vi "DAQ_System.vi"() -> ()   [LabVIEW 2023]
doc: "This is the Main VI that performs DAQ system and simulate the Same."
uses:
  Controls/DAQ Inputs.ctl
  Controls/DAQ_Output.ctl
  Controls/Queue_Operation_Select.ctl
  Controls/DAQ_Data.ctl
  Controls/Acquired_Data.ctl
  Controls/State_and_Data.ctl
  Controls/Notifier_Operation_Select.ctl
  Controls/Timer_Select.ctl
  Controls/Error_Data.ctl
panel:
  out "Error_Out":errorcluster
  in  "Error_In":errorcluster
  in  "Stop":bool
  out "DAQ_Output":T1
  in  "DAQ_Inputs":T2={"Digial_In"={"AC_Power_Supply"=FALSE}, "Analog_In"={"Power_Consumption"=0.0, "Battery_Power"=100.0}} caption="DAQ Inputs" {"Analog_In"."Battery_Power" scale=0.0..100.0; "Analog_In"."Power_Consumption" scale=0.0..10.0}
  # "DAQ Simulator"
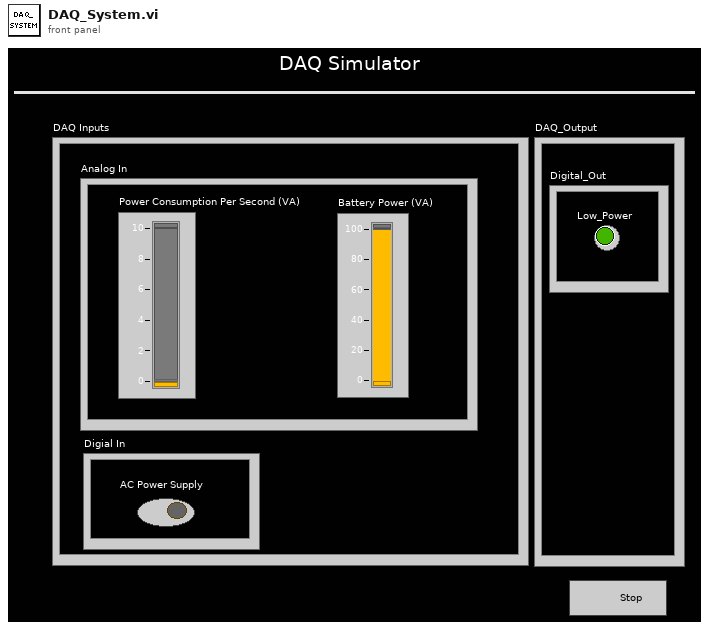
[diagram p1: front panel]
types:
  T1 = typedef "DAQ_Output.ctl" = cluster{"Digital_Out":cluster{"Low_Power":bool}}
  T2 = typedef "DAQ Inputs.ctl" = cluster{"Digial_In":cluster{"AC_Power_Supply":bool}, "Analog_In":cluster{"Power_Consumption":dbl, "Battery_Power":dbl}}
  T3 = typedef "State_and_Data.ctl" = cluster{"State":string, "Data":variant}
  T4 = typedef "Timer_Select.ctl" = enum16{"Start_Timer", "Time_Out?", "Stop_Timer"}
  T5 = typedef "Notifier_Operation_Select.ctl" = enum16{"Obtain_Notifier", "Send_Notification", "Get_Notifier_Status", "Release_Notifier"}
  T6 = typedef "Queue_Operation_Select.ctl" = enum16{"Obtain_Queue", "Enqueue", "Enqueue_First", "Enqueue_N", "Lossy_Enqueue", "Preview", "Queue_Status", "Dequeue", "Flush", "Release_Queue"}
  T7 = typedef "DAQ_Data.ctl" = cluster{"Acquired_Data":T8, "DAQ_Output":T1, "DAQ_Inputs":T2, "Data_In":T3, "Start":bool}
  T8 = typedef "Acquired_Data.ctl" = cluster{"Battery_Power":dbl, "Power_Consumption":dbl, "Inverter_Mode":bool}
  T9 = enum32{"Invalid", "Standard", "Closed", "Hidden", "Minimized", "Maximized"}
  T10 = typedef "Error_Data.ctl" = cluster{"Module_Name":string, "Error":errorcluster}
  T11 = cluster{"Power_Consumption":dbl, "Battery_Power":dbl}
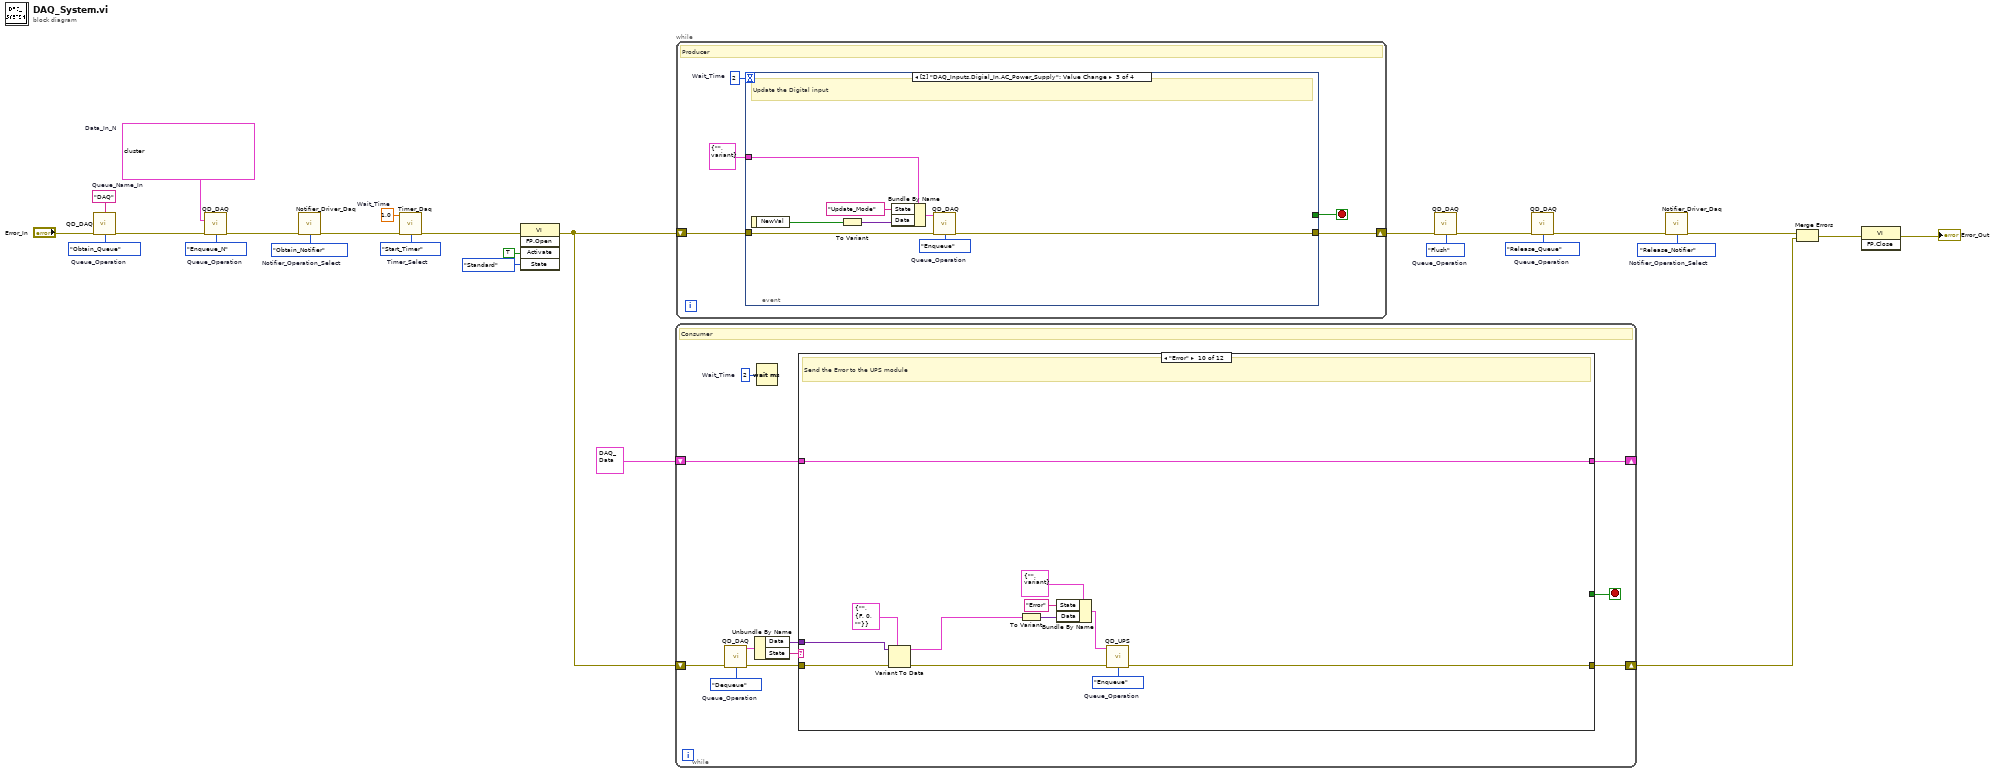
[diagram p0: block diagram]
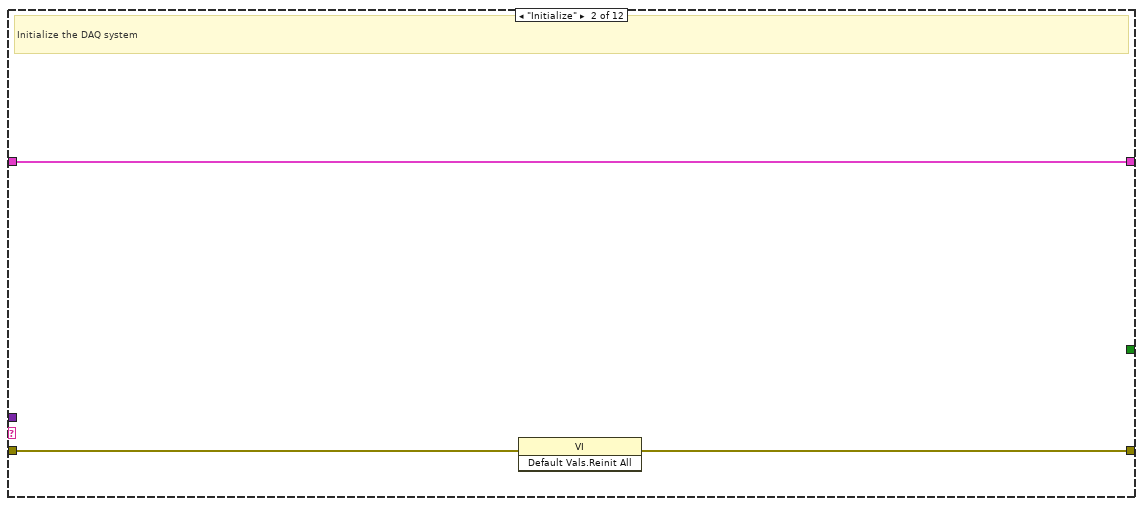
[diagram p3: hidden frame]
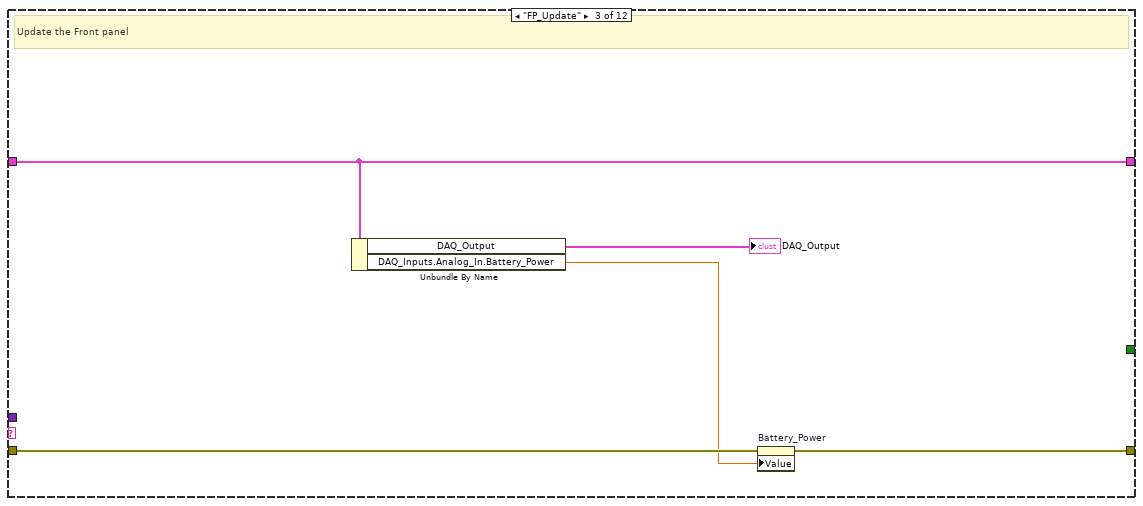
[diagram p4: hidden frame]
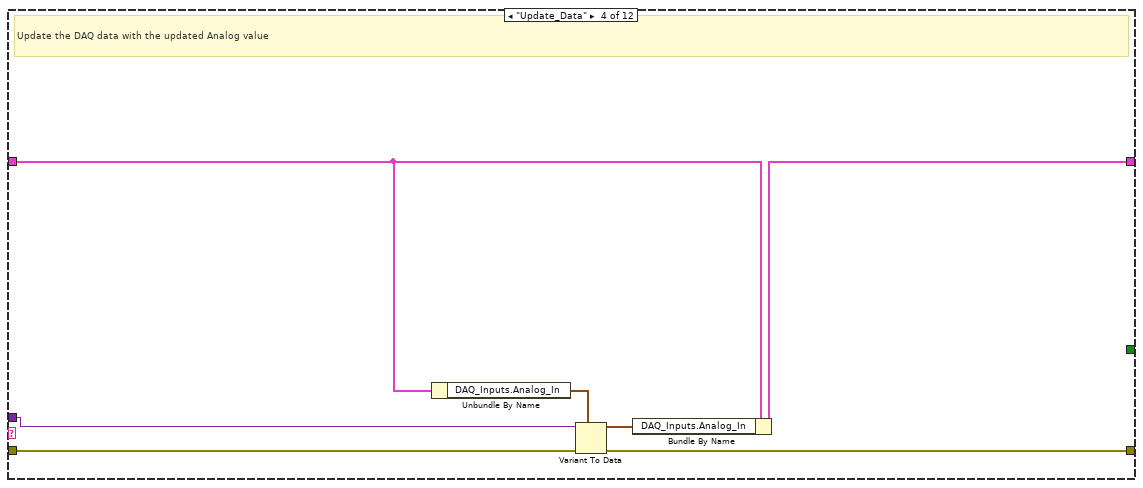
[diagram p5: hidden frame]
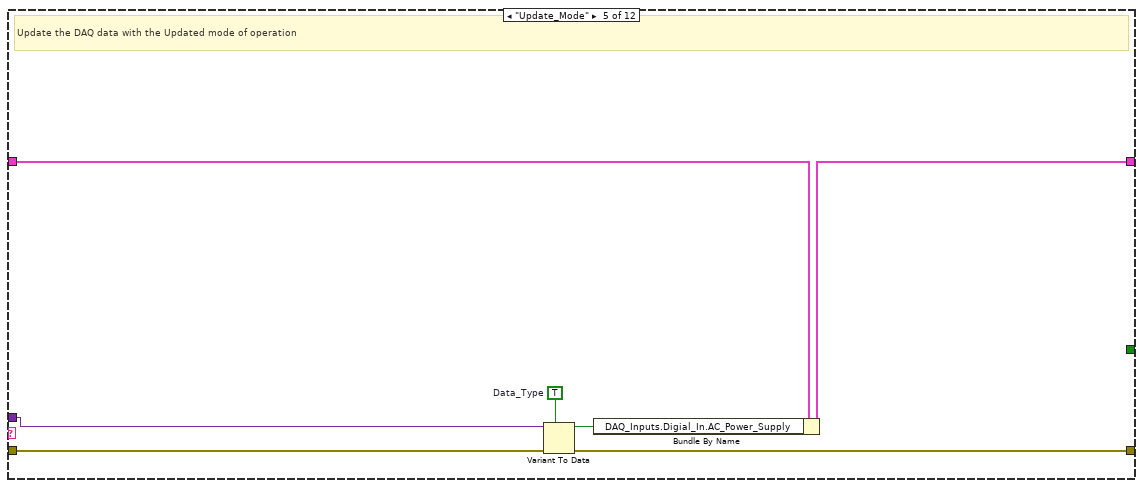
[diagram p6: hidden frame]
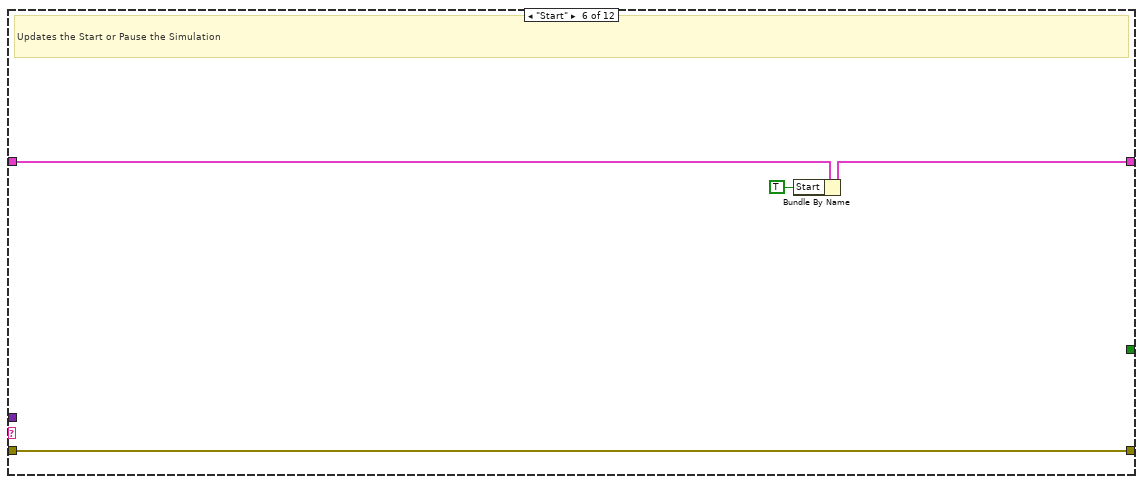
[diagram p7: hidden frame]
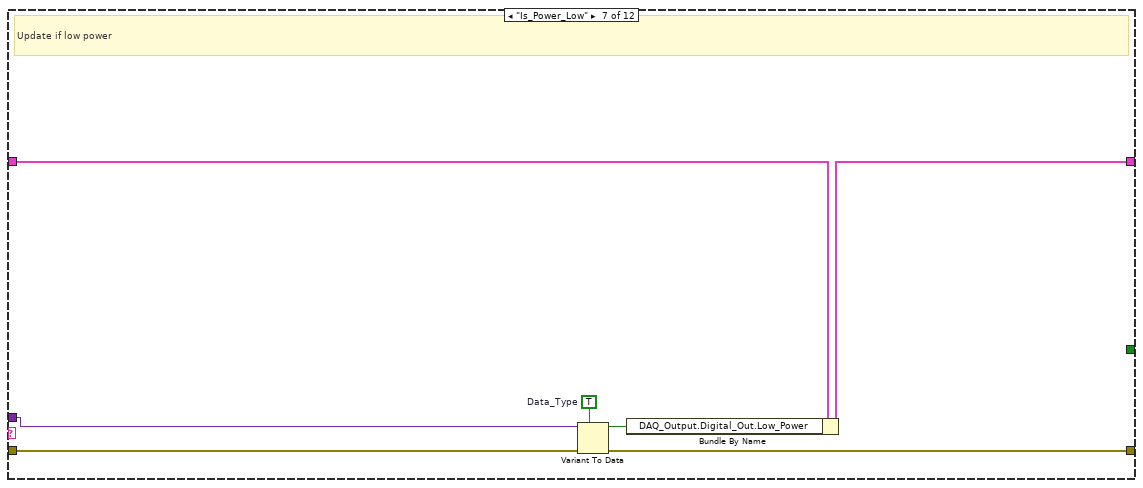
[diagram p8: hidden frame]
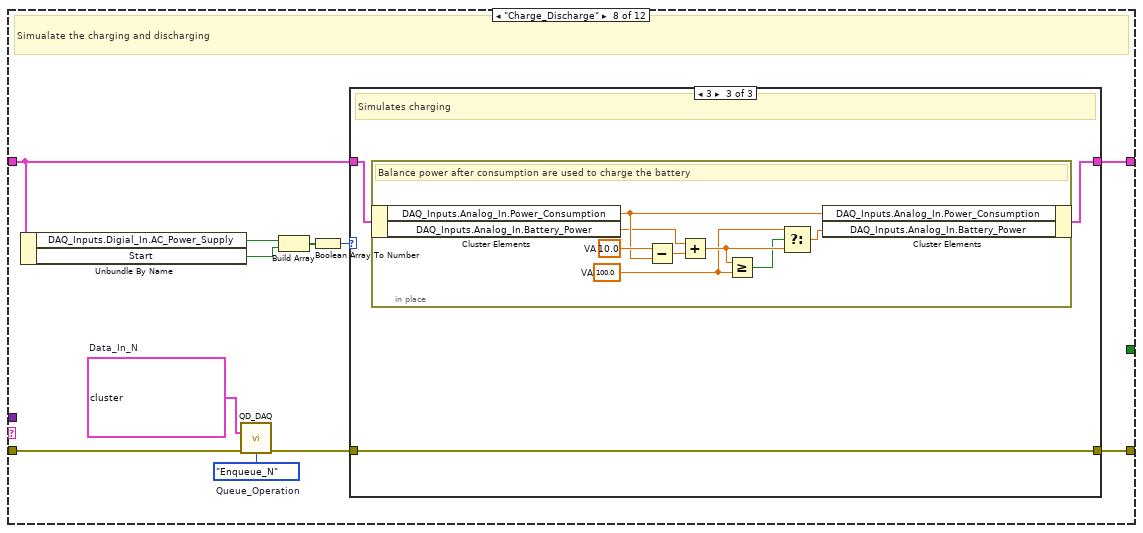
[diagram p9: hidden frame]
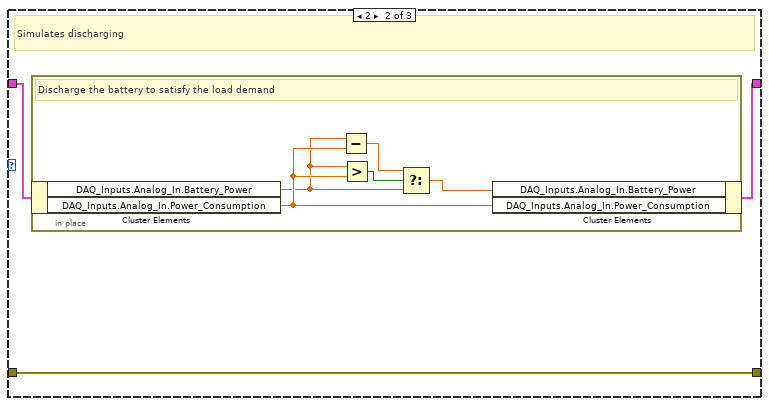
[diagram p11: hidden frame]
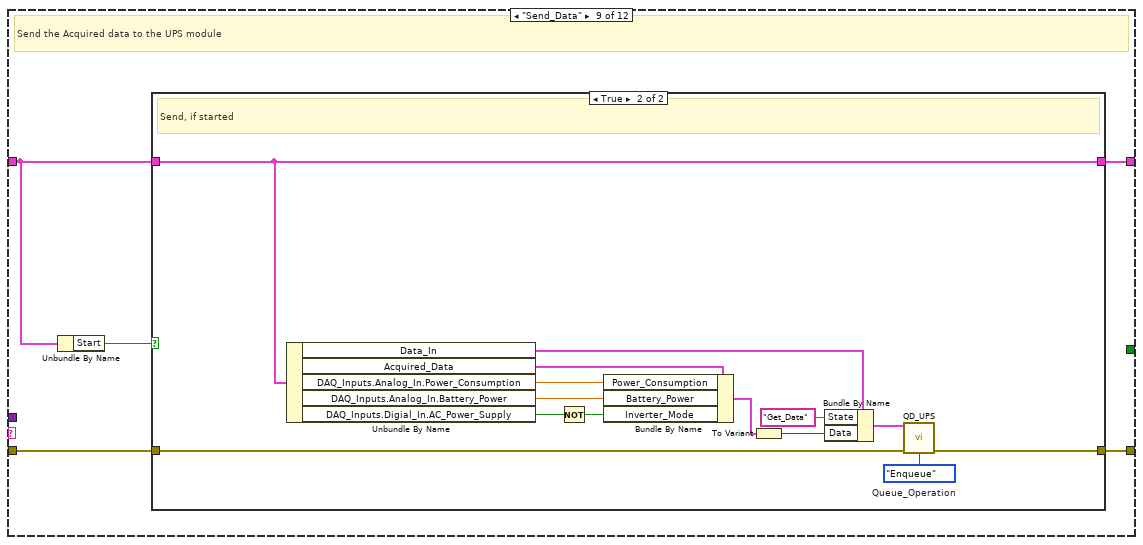
[diagram p12: hidden frame]
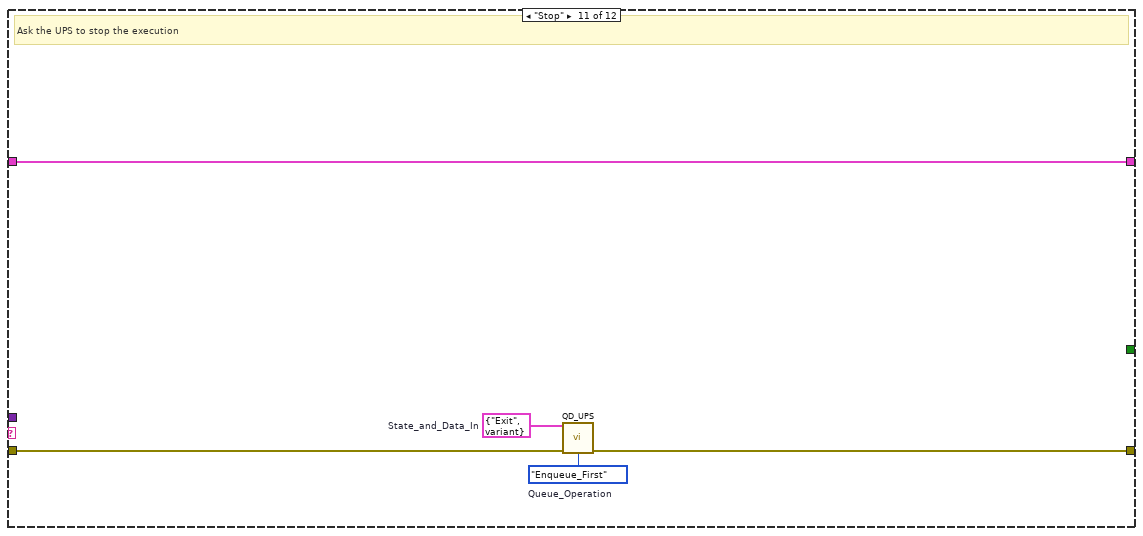
[diagram p14: hidden frame]
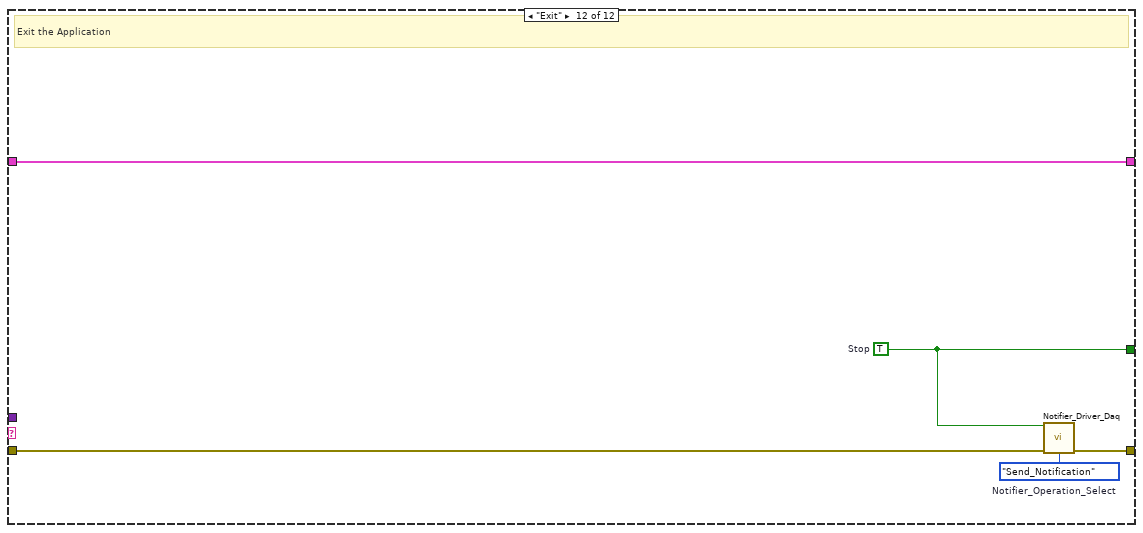
[diagram p15: hidden frame]
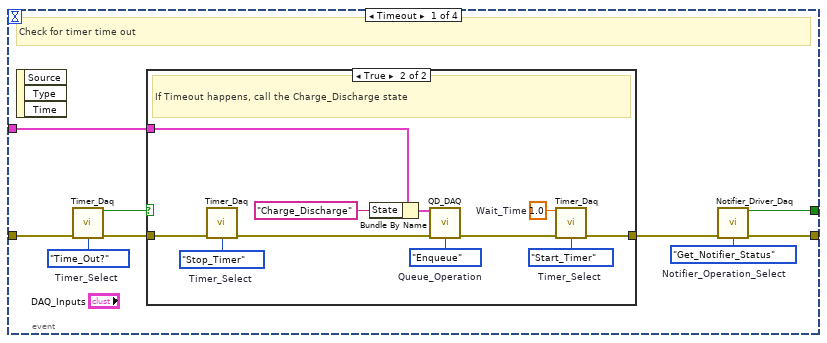
[diagram p16: hidden frame]
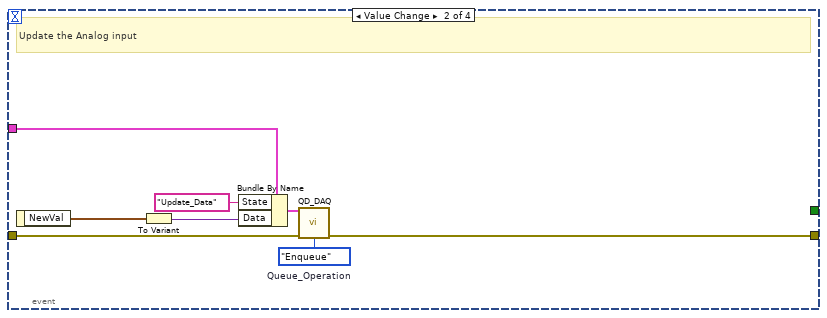
[diagram p18: hidden frame]
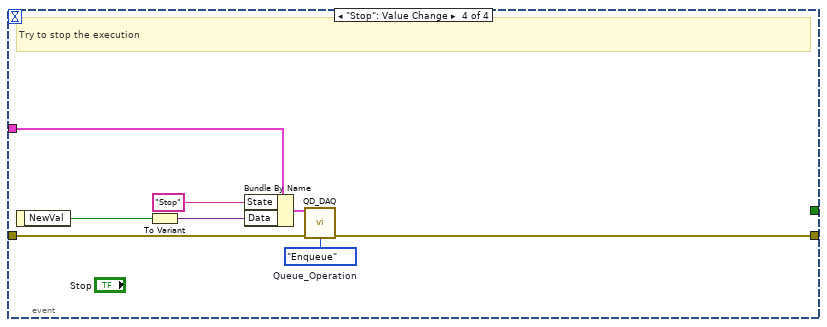
[diagram p19: hidden frame]
diagram:
  w1 = T3[] [{"State"="Initialize", "Data"=variant}, {"State"="Start", "Data"=variant}]  # Data_In_N
  w2 = 1.0  # Wait_Time
  w3 = Timer_Select."Start_Timer"  # Timer_Select
  w6 = Notifier_Operation_Select."Release_Notifier"  # Notifier_Operation_Select
  w8 = Notifier_Operation_Select."Obtain_Notifier"  # Notifier_Operation_Select
  w11 = Queue_Operation_Select."Enqueue_N"  # Queue_Operation
  w15 = Queue_Operation_Select."Release_Queue"  # Queue_Operation
  w17 = Queue_Operation_Select."Flush"  # Queue_Operation
  w19 = "DAQ"  # Queue_Name_In
  w24 = Queue_Operation_Select."Obtain_Queue"  # Queue_Operation
  n1 = call "QD_DAQ.vi"("Queue_Name_In"=w19, "Error_In"="Error_In", "Queue_Operation"=w24) -> ("Error_Out"=w25:errorcluster)  [unwired: 11 in, 1 out]
  n2 = call "QD_DAQ.vi"("Data_In_N"=w1, "Error_In"=w25, "Queue_Operation"=w11) -> ("Error_Out"=w12:errorcluster)  [unwired: 11 in, 1 out]
  n3 = call "Notifier_Driver_Daq.vi"("Error_In"=w12, "Notifier_Operation_Select"=w8) -> ("Error_Out"=w9:errorcluster)  [unwired: 12 in, 1 out]
  n4 = call "Timer_Daq.vi"("Wait_Time"=w2, "Error_In"=w9, "Timer_Select"=w3) -> ("Error_Out"=w4:errorcluster)  [unwired: 11 in, 1 out]
  n5 = invoke class="VI" method="FP.Open"(error in=w4, "Activate"=TRUE ("Activate?"), "State"=T9."Standard") -> (error out=w21:errorcluster)  [unwired: 2 in, 4 out]
  n6 = while {
    shift-right: [w31] -> _
    shift-left: T7 {"Acquired_Data"={"Battery_Power"=0.0, "Power_Consumption"=0.0, "Inverter_Mode"=FALSE}, "DAQ_Output"={"Digital_Out"={"Low_Power"=FALSE}}, "DAQ_Inputs"={"Digial_In"={"AC_Power_Supply"=FALSE}, "Analog_In"={"Power_Consumption"=0.0, "Battery_Power"=0.0}}, "Data_In"={"State"="", "Data"=variant}, "Start"=FALSE} -> [w30]
    shift-right: [w28] -> w13
    shift-left: w21 -> [w37]
    stop <- w29 stop-if-true
    w27 = u32 2  # Wait_Time
    w35 = Queue_Operation_Select."Dequeue"  # Queue_Operation
    # "Consumer"
    n7 = call "QD_DAQ.vi"("Error_In"=w37, "Queue_Operation"=w35) -> ("State_and_Data_Out"=w34:T3, "Error_Out"=w36:errorcluster)  [unwired: 12 in]
    n8 = Unbundle By Name(w34) -> ("Data"=w32:variant, "State"=w33:string)
    n9 = Wait (ms)(milliseconds to wait=w27) -> ()  [unwired: 1 out]
    n10 = case shown="\"Error\"" w33 {
      tunnel: w36 -> [w39 w42 w47 w54 w61 w63 w71 w74 w105 w130 w141 w146]
      tunnel: [w39 w41 w45 w53 w60 w63 w70 w77 w109 w137 w140 w145] -> w28
      tunnel: w32 -> [_ _ _ w52 w59 _ w69 _ _ w128 _ _]
      tunnel: [w38 w40 w46 w49 w56 w64 w67 w83 w108 w134 w142 w147] -> w31
      tunnel: w30 -> [w38 w40 w46 w50 w58 w65 w72 w82 w107 w134 w142 w147]
      tunnel: [_ _ _ _ _ _ _ _ _ _ _ w143] -> w29
      frame Default {
      }
      frame "Initialize" {
        # "Initialize the DAQ system"
        n11 = invoke class="VI" method="Default Vals.Reinit All"(error in=w42) -> (error out=w41:errorcluster)  [unwired: 2 in, 2 out]
      }
      frame "FP_Update" {
        # "Update the Front panel"
        n12 = Unbundle By Name(w46) -> ("DAQ_Output"=→"DAQ_Output":T1, "DAQ_Inputs.Analog_In.Battery_Power"=w44:dbl)
        n13 = property on="Battery_Power" class="Slide (strict)"(error in=w47, "Value"=w44) -> (error out=w45:errorcluster)  [unwired: 1 in, 1 out]
      }
      frame "Update_Data" {
        # "Update the DAQ data with the updated Analog value"
        n14 = Unbundle By Name(w50) -> ("DAQ_Inputs.Analog_In"=w51:T11)
        n15 = Variant To Data(error in=w54, type=w51, Variant=w52) -> (data=w48:T11, error out=w53:errorcluster)
        n16 = Bundle By Name(cluster=w50, "DAQ_Inputs.Analog_In"=w48) -> (w49:T7)
      }
      frame "Update_Mode" {
        w57 = TRUE  # Data_Type
        # "Update the DAQ data with the Updated mode of operation"
        n17 = Variant To Data(error in=w61, type=w57, Variant=w59) -> (data=w55:bool, error out=w60:errorcluster)
        n18 = Bundle By Name(cluster=w58, "DAQ_Inputs.Digial_In.AC_Power_Supply"=w55) -> (w56:T7)
      }
      frame "Start" {
        # "Updates the Start or Pause the Simulation"
        n19 = Bundle By Name(cluster=w65, "Start"=TRUE) -> (w64:T7)
      }
      frame "Is_Power_Low" {
        w68 = TRUE  # Data_Type
        # "Update if low power"
        n20 = Variant To Data(error in=w71, type=w68, Variant=w69) -> (data=w66:bool, error out=w70:errorcluster)
        n21 = Bundle By Name(cluster=w72, "DAQ_Output.Digital_Out.Low_Power"=w66) -> (w67:T7)
      }
      frame "Charge_Discharge" {
        w75 = T3[] [{"State"="Send_Data", "Data"=variant}, {"State"="FP_Update", "Data"=variant}]  # Data_In_N
        w76 = Queue_Operation_Select."Enqueue_N"  # Queue_Operation
        # "Simualate the charging and discharging"
        n22 = Unbundle By Name(w82) -> ("DAQ_Inputs.Digial_In.AC_Power_Supply"=w81:bool, "Start"=w80:bool)
        n23 = call "QD_DAQ.vi"("Data_In_N"=w75, "Error_In"=w74, "Queue_Operation"=w76) -> ("Error_Out"=w73:errorcluster)  [unwired: 11 in, 1 out]
        n24 = Build Array(w81, w80) -> (w79:bool[])
        n25 = Boolean Array To Number(Boolean array=w79) -> (number=w78:u32)
        n26 = case shown="3" w78 {
          tunnel: w73 -> [w84 w88 w96]
          tunnel: [w84 w88 w96] -> w77
          tunnel: w82 -> [w85 w87 w95]
          tunnel: [w85 w86 w94] -> w83
          frame 0, Default {
          }
          frame 2 {
            # "Simulates discharging"
            n27 = in-place {
              # "Discharge the battery to satisfy the load demand"
              n28 = in-place-cluster #1(w87) -> ("DAQ_Inputs.Analog_In.Battery_Power"=w89:dbl, "DAQ_Inputs.Analog_In.Power_Consumption"=w92:dbl)
              n29 = Subtract(x=w89, y=w92) -> (x-y=w93:dbl)
              n30 = Greater?(x=w89, y=w92) -> (0:w90:bool)
              n31 = Select(t=w93, s=w90, f=w89) -> (s? t:f=w91:dbl)
              n32 = in-place-cluster #1("DAQ_Inputs.Analog_In.Battery_Power"=w91, "DAQ_Inputs.Analog_In.Power_Consumption"=w92) -> (w86:T7)
            }
          }
          frame 3 {
            # "Simulates charging"
            n33 = in-place {
              w97 = 100.0  # VA
              w103 = 10.0  # VA
              # "Balance power after consumption are used to charge the battery"
              n34 = in-place-cluster #2(w95) -> ("DAQ_Inputs.Analog_In.Power_Consumption"=w102:dbl, "DAQ_Inputs.Analog_In.Battery_Power"=w99:dbl)
              n35 = Subtract(x=w103, y=w102) -> (x-y=w101:dbl)
              n36 = Add(x=w99, y=w101) -> (x+y=w100:dbl)
              n37 = Greater Or Equal?(x=w100, y=w97) -> (x >= y?=w98:bool)
              n38 = Select(t=w97, s=w98, f=w100) -> (s? t:f=w104:dbl)
              n39 = in-place-cluster #2("DAQ_Inputs.Analog_In.Power_Consumption"=w102, "DAQ_Inputs.Analog_In.Battery_Power"=w104) -> (w94:T7)
            }
          }
        }
      }
      frame "Send_Data" {
        # "Send the Acquired data to the UPS module"
        n40 = Unbundle By Name(w107) -> ("Start"=w106:bool)
        n41 = case shown="True" w106 {
          tunnel: w105 -> [w110 w114]
          tunnel: [w110 w113] -> w109
          tunnel: [w111 w121] -> w108
          tunnel: w107 -> [w111 w121]
          frame False {
          }
          frame True {
            w125 = Queue_Operation_Select."Enqueue"  # Queue_Operation
            # "Send, if started"
            n42 = Unbundle By Name(w121) -> ("Data_In"=w120:T3, "Acquired_Data"=w119:T8, "DAQ_Inputs.Analog_In.Power_Consumption"=w118:dbl, "DAQ_Inputs.Analog_In.Battery_Power"=w117:dbl, "DAQ_Inputs.Digial_In.AC_Power_Supply"=w116:bool)
            n43 = Not(x=w116) -> (.not. x?=w112:bool)
            n44 = Bundle By Name(cluster=w119, "Power_Consumption"=w118, "Battery_Power"=w117, "Inverter_Mode"=w112) -> (w115:T8)
            n45 = To Variant(anything=w115) -> (Variant=w123:variant)
            n46 = Bundle By Name(cluster=w120, "State"="Get_Data", "Data"=w123) -> (w124:T3)
            n47 = call "QD_UPS.vi"("State_and_Data_In"=w124, "Error_In"=w114, "Queue_Operation"=w125) -> ("Error_Out"=w113:errorcluster)  [unwired: 11 in, 1 out]
          }
        }
      }
      frame "Error" {
        w136 = Queue_Operation_Select."Enqueue"  # Queue_Operation
        # "Send the Error to the UPS module"
        n48 = Variant To Data(error in=w130, type=T10 {"Module_Name"="", "Error"={"status"=FALSE, "code"=0, "source"=""}} ("Error_Data"), Variant=w128) -> (data=w126:T10, error out=w129:errorcluster)
        n49 = To Variant(anything=w126) -> (Variant=w131:variant)
        n50 = Bundle By Name(cluster=T3 {"State"="", "Data"=variant} ("State_and_Data"), "State"="Error", "Data"=w131) -> (w135:T3)
        n51 = call "QD_UPS.vi"("State_and_Data_In"=w135, "Error_In"=w129, "Queue_Operation"=w136) -> ("Error_Out"=w137:errorcluster)  [unwired: 11 in, 1 out]
      }
      frame "Stop" {
        w138 = T3 {"State"="Exit", "Data"=variant}  # State_and_Data_In
        w139 = Queue_Operation_Select."Enqueue_First"  # Queue_Operation
        # "Ask the UPS to stop the execution"
        n52 = call "QD_UPS.vi"("State_and_Data_In"=w138, "Error_In"=w141, "Queue_Operation"=w139) -> ("Error_Out"=w140:errorcluster)  [unwired: 11 in, 1 out]
      }
      frame "Exit" {
        w144 = Notifier_Operation_Select."Send_Notification"  # Notifier_Operation_Select
        w143 = TRUE  # Stop
        # "Exit the Application"
        n53 = call "Notifier_Driver_Daq.vi"("Notification"=w143, "Error_In"=w146, "Notifier_Operation_Select"=w144) -> ("Error_Out"=w145:errorcluster)  [unwired: 11 in, 1 out]
      }
    }
  }
  n54 = while {
    shift-right: [w148] -> w5
    shift-left: w21 -> [w152]
    stop <- w151 stop-if-true
    w150 = 2  # Wait_Time
    # "Producer"
    n55 = event shown="[2] \"DAQ_Inputs.Digial_In.AC_Power_Supply\": Value Change" {
      selector: _ -> [_ _ _ _]
      dyn-events: _ -> [_ _ _ _]
      timeout: w150 -> [_ _ _ _]
      tunnel: w152 -> [w161 w176 w183 w195]
      tunnel: [w159 _ _ _] -> w151
      tunnel: [w158 w175 w184 w194] -> w148
      tunnel: T3 {"State"="", "Data"=variant} ("Data_In") -> [w154 w174 w182 w192]
      event Timeout {
        w155 = Timer_Select."Time_Out?"  # Timer_Select
        w160 = Notifier_Operation_Select."Get_Notifier_Status"  # Notifier_Operation_Select
        # "Check for timer time out"
        n56 = event-data() -> ()  [unwired: 1 in, 3 out]
        n57 = call "Timer_Daq.vi"("Error_In"=w161, "Timer_Select"=w155) -> ("Time_Out?"=w153:bool, "Error_Out"=w157:errorcluster)  [unwired: 12 in]
        n58 = case shown="True" w153 {
          tunnel: w157 -> [w162 w173]
          tunnel: [w162 w170] -> w156
          tunnel: w154 -> [_ w166]
          frame False {
          }
          frame True {
            w163 = 1.0  # Wait_Time
            w167 = Timer_Select."Start_Timer"  # Timer_Select
            w168 = Queue_Operation_Select."Enqueue"  # Queue_Operation
            w169 = Timer_Select."Stop_Timer"  # Timer_Select
            # "If Timeout happens, call the Charge_Discharge state"
            n59 = call "Timer_Daq.vi"("Error_In"=w173, "Timer_Select"=w169) -> ("Error_Out"=w172:errorcluster)  [unwired: 12 in, 1 out]
            n60 = Bundle By Name(cluster=w166, "State"="Charge_Discharge") -> (w165:T3)
            n61 = call "QD_DAQ.vi"("State_and_Data_In"=w165, "Error_In"=w172, "Queue_Operation"=w168) -> ("Error_Out"=w171:errorcluster)  [unwired: 11 in, 1 out]
            n62 = call "Timer_Daq.vi"("Wait_Time"=w163, "Error_In"=w171, "Timer_Select"=w167) -> ("Error_Out"=w170:errorcluster)  [unwired: 11 in, 1 out]
          }
        }
        n63 = call "Notifier_Driver_Daq.vi"("Error_In"=w156, "Notifier_Operation_Select"=w160) -> ("Latest_Notification"=w159:bool, "Error_Out"=w158:errorcluster)  [unwired: 12 in]
      }
      event Value Change {
        w179 = Queue_Operation_Select."Enqueue"  # Queue_Operation
        # "Update the Analog input"
        n64 = event-data() -> ("NewVal"=w181:T11)  [unwired: 1 in]
        n65 = To Variant(anything=w181) -> (Variant=w178:variant)
        n66 = Bundle By Name(cluster=w174, "State"="Update_Data", "Data"=w178) -> (w180:T3)
        n67 = call "QD_DAQ.vi"("State_and_Data_In"=w180, "Error_In"=w176, "Queue_Operation"=w179) -> ("Error_Out"=w175:errorcluster)  [unwired: 11 in, 1 out]
      }
      event Value Change {
        w187 = Queue_Operation_Select."Enqueue"  # Queue_Operation
        # "Update the Digital input"
        n68 = event-data() -> ("NewVal"=w189:bool)  [unwired: 1 in]
        n69 = To Variant(anything=w189) -> (Variant=w185:variant)
        n70 = Bundle By Name(cluster=w182, "State"="Update_Mode", "Data"=w185) -> (w188:T3)
        n71 = call "QD_DAQ.vi"("State_and_Data_In"=w188, "Error_In"=w183, "Queue_Operation"=w187) -> ("Error_Out"=w184:errorcluster)  [unwired: 11 in, 1 out]
      }
      event "Stop": Value Change {
        w196 = Queue_Operation_Select."Enqueue"  # Queue_Operation
        # "Try to stop the execution"
        n72 = event-data() -> ("NewVal"=w191:bool)  [unwired: 1 in]
        n73 = To Variant(anything=w191) -> (Variant=w190:variant)
        n74 = Bundle By Name(cluster=w192, "State"="Stop", "Data"=w190) -> (w197:T3)
        n75 = call "QD_DAQ.vi"("State_and_Data_In"=w197, "Error_In"=w195, "Queue_Operation"=w196) -> ("Error_Out"=w194:errorcluster)  [unwired: 11 in, 1 out]
      }
    }
  }
  n76 = call "QD_DAQ.vi"("Error_In"=w5, "Queue_Operation"=w17) -> ("Error_Out"=w18:errorcluster)  [unwired: 12 in, 1 out]
  n77 = call "QD_DAQ.vi"("Error_In"=w18, "Queue_Operation"=w15) -> ("Error_Out"=w16:errorcluster)  [unwired: 12 in, 1 out]
  n78 = call "Notifier_Driver_Daq.vi"("Error_In"=w16, "Notifier_Operation_Select"=w6) -> ("Error_Out"=w7:errorcluster)  [unwired: 12 in, 1 out]
  n79 = Merge Errors(w7, w13) -> (w14:errorcluster)
  n80 = invoke class="VI" method="FP.Close"(error in=w14) -> (error out=→"Error_Out":errorcluster)  [unwired: 2 in, 2 out]
